vi "Play Sound.vi"(8 "error in (no error)":errorcluster, 11 "Sound":waveform(dbl)={"t0"=timestamp(0 s since 1904-01-01), "dt"=0.0, "Y"=[]}) -> (0 "error out":errorcluster)   [LabVIEW 2018]
uses:
  <vilib>/sound2/lvsound2.llb/Sound Data Format.ctl
  <vilib>/sound2/lvsound2.llb/Sound Output Write (DBL Single).vi
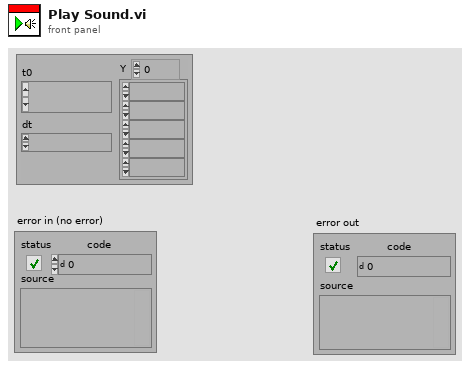
[diagram p1: front panel]
types:
  T1 = typedef "Sound Data Format.ctl" = cluster{"sample rate (S/s)":dbl, "number of channels":i32, "bits per sample":i32}
  T2 = typedef "Sound Output Task ID.ctl" = u32
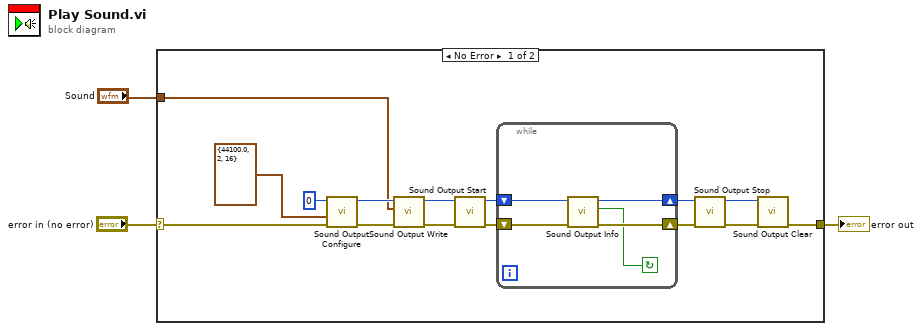
[diagram p0: block diagram]
diagram:
  n1 = case shown="No Error" "error in (no error)" {
    selector: "error in (no error)" -> [w8 w24]
    tunnel: [w5 w24] -> w2
    tunnel: "Sound" -> [w4 _]
    frame No Error {
      n2 = call <vilib>:"Sound Output Configure.vi"("error in (no error)"=w8, "sound format"=T1 {"sample rate (S/s)"=44100.0, "number of channels"=2, "bits per sample"=16}, "device ID"=u32 0) -> ("error out"=w16:errorcluster, "task ID"=w17:T2)  [unwired: 7 in]
      n3 = call-poly <vilib>:"Sound Output Write.vi"("error in (no error)"=w16, "data"=w4, "task ID"=w17) -> ("error out"=w14:errorcluster, "task ID out"=w15:T2)  [unwired: 7 in]
      n4 = call <vilib>:"Sound Output Start.vi"("error in (no error)"=w14, "task ID"=w15) -> ("error out"=w12:errorcluster, "task ID out"=w13:T2)  [unwired: 8 in]
      n5 = while {
        shift-right: [w21] -> w11
        shift-left: w13 -> [w23]
        shift-right: [w20] -> w10
        shift-left: w12 -> [w22]
        stop <- w19 continue-if-true
        n6 = call <vilib>:"Sound Output Info.vi"("error in (no error)"=w22, "task ID"=w23) -> ("error out"=w20:errorcluster, "is playing?"=w19:bool, "task ID out"=w21:T2)  [unwired: 6 in, 1 out]
      }
      n7 = call <vilib>:"Sound Output Stop.vi"("error in (no error)"=w10, "task ID"=w11) -> ("error out"=w6:errorcluster, "task ID out"=w7:T2)  [unwired: 8 in]
      n8 = call <vilib>:"Sound Output Clear.vi"("error in (no error)"=w6, "task ID"=w7) -> ("error out"=w5:errorcluster)  [unwired: 9 in]
    }
    frame Error {
    }
  }
  "error out" <- w2
